vi "SDSU_Numb2Dec.vi"(10 "input str":string) -> (1 "output hexa":string, 2 "remaining string":string, 3 "hexa?":bool)   [LabVIEW 2016]
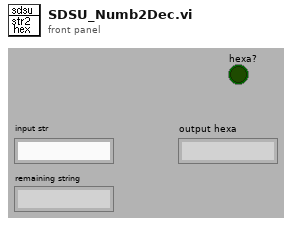
[diagram p1: front panel]
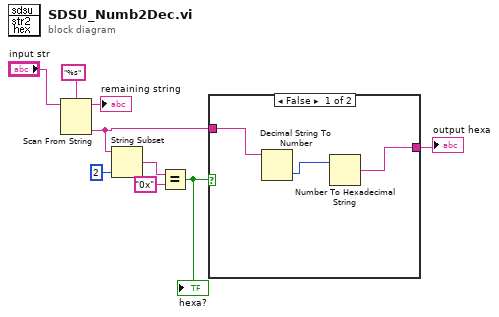
[diagram p0: block diagram]
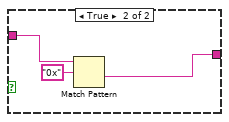
[diagram p2: hidden frame]
diagram:
  n1 = Scan From String(format string="%s", input string="input str") -> (remaining string=→"remaining string":string, output 1=w3:string)  [unwired: 2 in, 3 out]
  n2 = String Subset(string=w3, length (rest)=2 ("length (rest)")) -> (substring=w6:string)  [unwired: 1 out]
  n3 = Equal?(x=w6, y="0x") -> (x = y?=w4:bool)
  "hexa?" <- w4
  n4 = case shown="False" w4 {
    tunnel: w3 -> [w12 w15]
    tunnel: [w10 w13] -> w2
    frame False {
      n5 = Decimal String To Number(string=w12) -> (number=w11:i32)  [unwired: 3 out]
      n6 = Number To Hexadecimal String(2:w11) -> (0:w10:string)  [unwired: 1 out]
    }
    frame True {
      n7 = Match Pattern(string=w15, regular expression="0x") -> (after substring=w13:string)  [unwired: 4 out]
    }
  }
  "output hexa" <- w2
